vi "Stop All.vi"(8 "error in (no error)":errorcluster, 11 "LINX-PCA9865 PWM in":refnum<class "LINX-PCA9865 PWM.lvclass">) -> (0 "error out":errorcluster, 3 "LINX-PCA9865 PWM out":refnum<class "LINX-PCA9865 PWM.lvclass">)   [LabVIEW 2019, in "LINX-PCA9865 PWM.lvclass"]
uses:
  LINX-PCA9865 PWM.lvclass
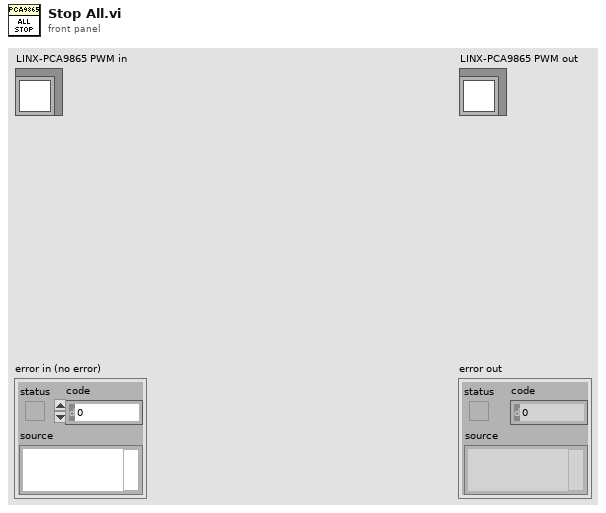
[diagram p1: front panel]
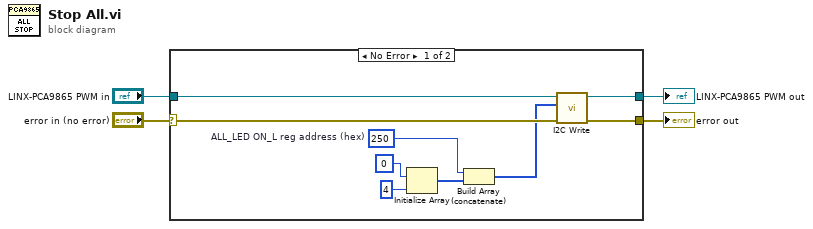
[diagram p0: block diagram]
diagram:
  n1 = case shown="No Error" "error in (no error)" {
    selector: "error in (no error)" -> [w13 w15]
    tunnel: [w12 w15] -> w3
    tunnel: [w10 w14] -> w1
    tunnel: "LINX-PCA9865 PWM in" -> [w11 w14]
    frame No Error {
      w8 = u8 250  # ALL_LED ON_L reg address (hex)
      n2 = Initialize Array(u8 0 ("I2C Slave Address 2"), 4 ("dimension size")) -> (w5:u8[])
      n3 = Build Array (concatenate)(w8, w5) -> (w9:u8[])
      n4 = call "I2C Write.vi"("error in (no error)"=w13, "Bytes to Write"=w9, "LINX-PCA9865 PWM in"=w11) -> ("error out"=w12:errorcluster, "LINX-PCA9865 PWM out"=w10:refnum<class "LINX-PCA9865 PWM.lvclass">)  [unwired: 7 in]
    }
    frame Error {
    }
  }
  "error out" <- w3
  "LINX-PCA9865 PWM out" <- w1
